vi "Query Marker Reflection Measurement.vi"(8 "error in (no error)":errorcluster, 10 "Active Marker (1: Marker 1)":i32(ring)=1 items=["Marker 1"=1, "Marker 2"=2, "Marker 3"=3, "Marker 4"=4, "Marker 5"=5, "Marker 6"=6], 11 "VISA resource name":refnum<visa-resource-name>) -> (0 "error out":errorcluster, 1 "Y Value":dbl, 2 "X Value":dbl, 3 "VISA resource name out":refnum<visa-resource-name>)   [LabVIEW 2022 SP3, in "Agilent N934X Series.lvlib"]
doc: "Query the marker value in Reflection Measurement measurement.\n\nNote:\nThis VI is only applicable for N9321C, N9322C, N9323C, N9324C models."
uses:
  <instrlib>/Agilent N934X Series/Agilent N934X Series.lvlib
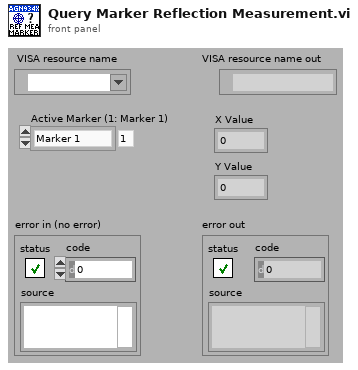
[diagram p1: front panel]
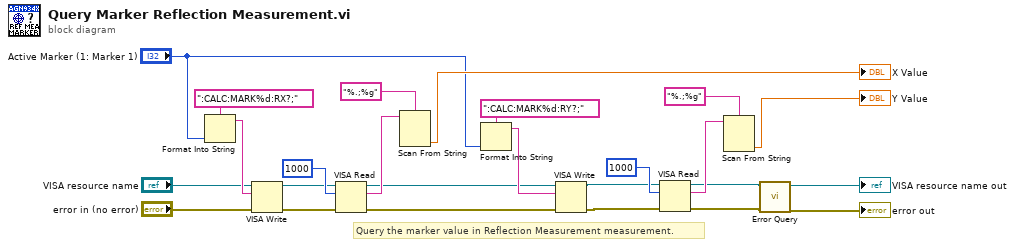
[diagram p0: block diagram]
diagram:
  # "Query the marker value in Reflection Measurement measurement."
  n1 = Format Into String(format string=":CALC:MARK%d:RX?;", "Active Marker (1: Marker 1)") -> (resulting string=w10:string)  [unwired: 2 in, 1 out]
  n2 = VISA Write(VISA resource name="VISA resource name", write buffer=w10, error in (no error)="error in (no error)") -> (VISA resource name out=w7:refnum<visa-resource-name>, error out=w6:errorcluster)  [unwired: 1 out]
  n3 = VISA Read(VISA resource name=w7, byte count=u32 1000, error in (no error)=w6) -> (VISA resource name out=w5:refnum<visa-resource-name>, read buffer=w12:string, error out=w4:errorcluster)  [unwired: 1 out]
  n4 = Scan From String(format string="%.;%g", input string=w12) -> (output 1=→"X Value":dbl)  [unwired: 3 in, 3 out]
  n5 = Format Into String(format string=":CALC:MARK%d:RY?;", "Active Marker (1: Marker 1)") -> (resulting string=w23:string)  [unwired: 2 in, 1 out]
  n6 = VISA Write(VISA resource name=w5, write buffer=w23, error in (no error)=w4) -> (VISA resource name out=w18:refnum<visa-resource-name>, error out=w17:errorcluster)  [unwired: 1 out]
  n7 = VISA Read(VISA resource name=w18, byte count=u32 1000, error in (no error)=w17) -> (VISA resource name out=w15:refnum<visa-resource-name>, read buffer=w19:string, error out=w16:errorcluster)  [unwired: 1 out]
  n8 = Scan From String(format string="%.;%g", input string=w19) -> (output 1=→"Y Value":dbl)  [unwired: 3 in, 3 out]
  n9 = call <instrlib>:"Error Query.vi"("error in (no error)"=w16, "VISA resource name"=w15) -> ("error out"=→"error out":errorcluster, "VISA resource name out"=→"VISA resource name out":refnum<visa-resource-name>)  [unwired: 6 in, 2 out]
